vi "Wave Manager.vi"(10 "Input Array":waveform(dbl)[](array[waveform]), 11 "data":waveform(dbl)) -> (2 "Waveform Graph Array":waveform(dbl)[](array[waveform]), 3 "Most Recent":dbl)   [LabVIEW 2016]
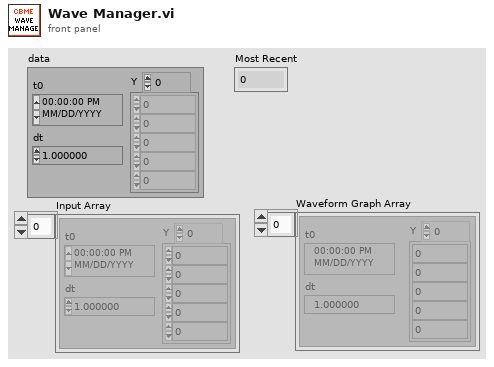
[diagram p1: front panel]
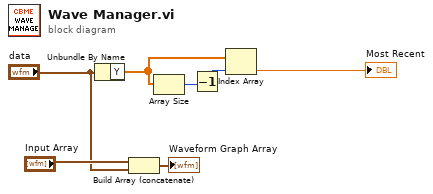
[diagram p0: block diagram]
diagram:
  n1 = Unbundle By Name("data") -> ("Y"=w6:dbl[])
  n2 = Build Array (concatenate)("Input Array", "data") -> (→"Waveform Graph Array":waveform(dbl)[])
  n3 = Array Size(array=w6) -> (size(s)=w4:i32)
  n4 = Decrement(x=w4) -> (x-1=w5:i32)
  n5 = Index Array(array=w6, index=w5) -> (element=→"Most Recent":dbl)
